vi "Get_cluster_element_by_name.vi"(2 "Label.Text":string, 3 "Controls[]":refnum<vi>[](array[refnum])) -> (0 "MatchedRefNum":bool, 1 "Ctl Refnum":refnum<vi>)   [LabVIEW 2011]
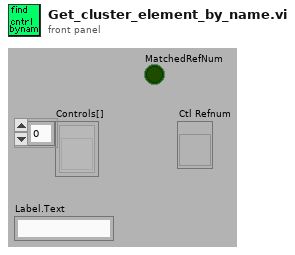
[diagram p1: front panel]
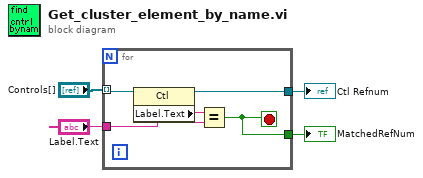
[diagram p0: block diagram]
diagram:
  n1 = for {
    tunnel: "Controls[]" -> [w9] mode=indexing
    tunnel: [w7] -> w2
    tunnel: "Label.Text" -> [w6]
    tunnel: [w5] -> w1
    stop <- w5 stop-if-true
    n2 = property class="Ctl"(reference=w9) -> (reference out=w7:refnum<vi>, "Label.Text"=w8:string)  [unwired: 1 in, 1 out]
    n3 = Equal?(x=w8, y=w6) -> (x = y?=w5:bool)
  }
  "Ctl Refnum" <- w2
  "MatchedRefNum" <- w1
